vi "Timer Setup.vi"(5 "Timers":T1={"Timer"={"Sun"=FALSE, "Timer"=FALSE, "Altitude"=0.0, "Action Time"=55500.0, "Mon"=FALSE, "Tues"=TRUE, "Wed"=FALSE, "Thur"=FALSE, "Fri"=FALSE, "Sat"=FALSE, "Mode"=enum."Run"}, "Timer 2"={"Sun"=FALSE, "Timer"=FALSE, "Altitude"=0.0, "Action Time"=55560.0, "Mon"=FALSE, "Tues"=TRUE, "Wed"=FALSE, "Thur"=FALSE, "Fri"=FALSE, "Sat"=FALSE, "Mode"=enum."Stby"}, "Timer 3"={"Sun"=FALSE, "Timer"=FALSE, "Altitude"=0.0, "Action Time"=55680.0, "Mon"=FALSE, "Tues"=TRUE, "Wed"=FALSE, "Thur"=FALSE, "Fri"=FALSE, "Sat"=FALSE, "Mode"=enum."Run"}, "Timer 4"={"Sun"=FALSE, "Timer"=FALSE, "Altitude"=0.0, "Action Time"=55740.0, "Mon"=FALSE, "Tues"=TRUE, "Wed"=FALSE, "Thur"=FALSE, "Fri"=FALSE, "Sat"=FALSE, "Mode"=enum."Off"}} {"Timer 4"."Action Time" format="%<%H:%M>t"; "Timer 3"."Action Time" format="%<%H:%M>t"; "Timer 2"."Action Time" format="%<%H:%M>t"; "Timer"."Action Time" format="%<%H:%M>t"}) -> ()   [LabVIEW 2012]
uses:
  Type Defs/All Timers.ctl
  Type Defs/Timer Control.ctl
  Altitude/Altitude.xctl
  Type Defs/Action Time.ctl
  Mode Control/Mode.xctl
  Scheduler/Builder/Schedule Builder.lvclass
  Scheduler/Configuration Data/Task Data.lvclass
  MSR/Sequence Composition/Sequence Factory/Sequence Builder.lvclass/Sequence Builder.ctl
  Scheduler/Builder/Schedule Builder.lvclass/Schedule Builder.ctl
  MSR/Sequence Composition/SEQ/SEQ.lvclass
  Scheduler/Scheduler SEQ/Scheduler.lvclass
  Scheduler/Scheduler SEQ/Scheduler.lvclass/Scheduler.ctl
  Scheduler/Scheduler SEQ/Write DOW.vi
  MSR/Sequence Composition/Sequence Factory/Sequence Builder.lvclass
panel:
  in  "Tab Control":enum32{"Page 1", "Page 2"}(tab)
  out "Messages":string[](array[string])
  out "Timer.Mode":enum8{"Off", "Stby", "Hold", "Run"}(ring)
  out "Timer.Altitude":sgl
  # "1"
  # "1"
  # "1"
  # "1"
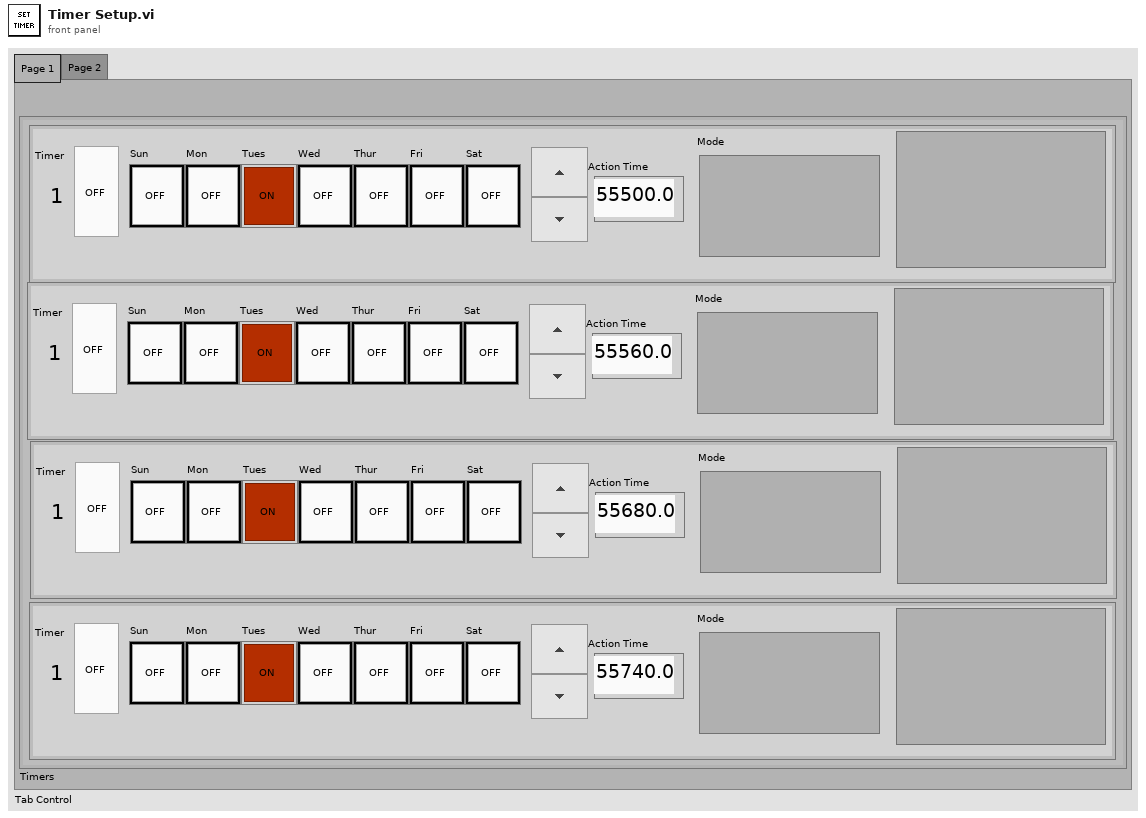
[diagram p1: front panel]
types:
  T1 = typedef "All Timers.ctl" = cluster{"Timer":T2, "Timer 2":T2, "Timer 3":T2, "Timer 4":T2}
  T2 = typedef "Timer Control.ctl" = cluster{"Sun":bool, "Timer":bool, "Altitude":sgl, "Action Time":T3, "Mon":bool, "Tues":bool, "Wed":bool, "Thur":bool, "Fri":bool, "Sat":bool, "Mode":enum8{"Off", "Stby", "Hold", "Run"}}
  T3 = typedef "Action Time.ctl" = dbl
  T4 = typedef "LVDateTimeRec.ctl" = cluster{"fractional second":dbl, "second":i32, "minute":i32, "hour":i32, "day of month":i32, "month":i32, "year":i32, "day of week":i32, "day of year":i32, "DST":i32}
  T5 = typedef "Mode Select.ctl" = enum8{"Off", "Stby", "Hold", "Run"}
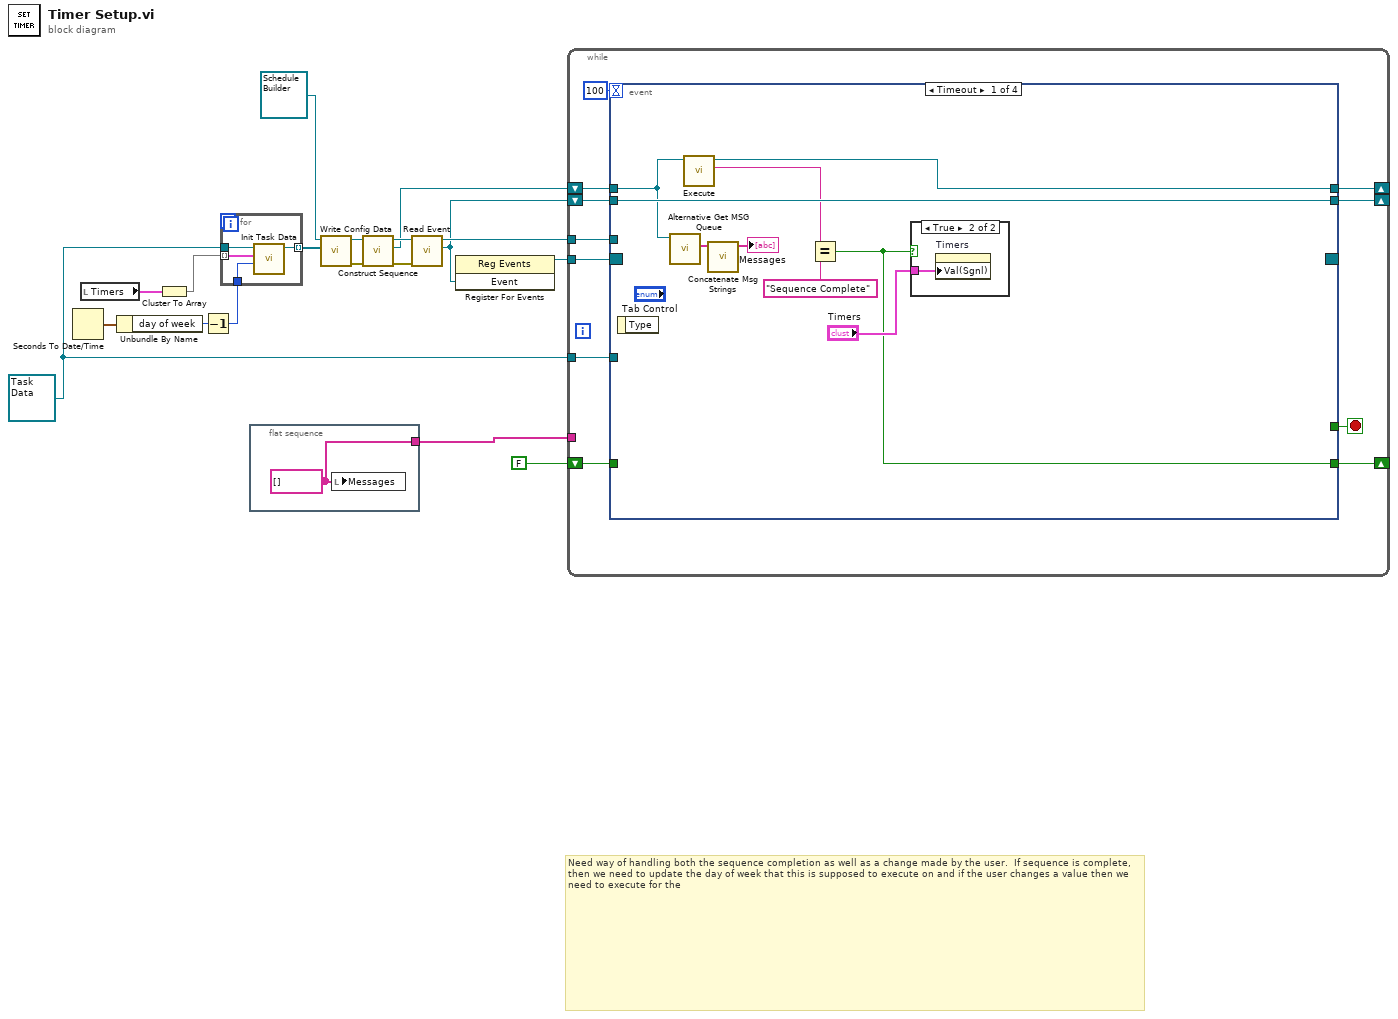
[diagram p0: block diagram]
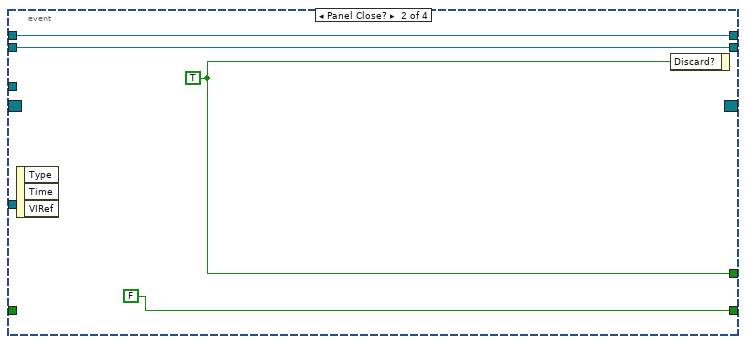
[diagram p3: hidden frame]
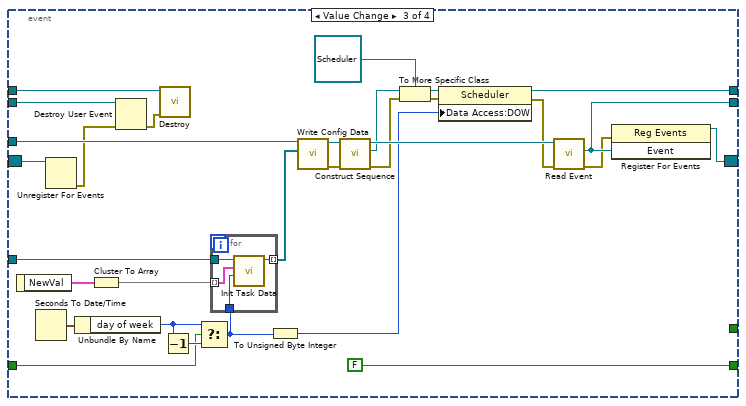
[diagram p4: hidden frame]
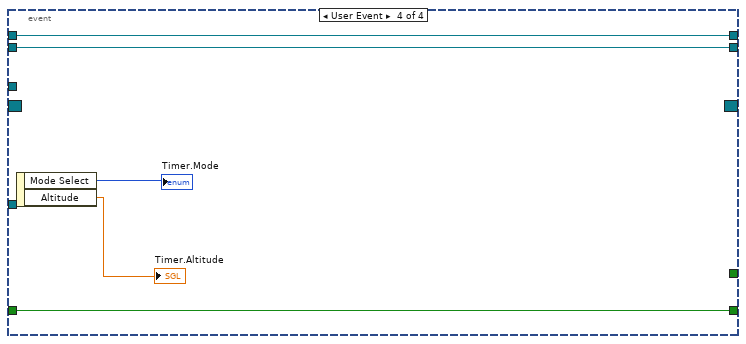
[diagram p5: hidden frame]
diagram:
  w8 = refnum<class "Task Data.lvclass"> refnum ("Task Data")
  # "Need way of handling both the sequence completion as well as a change made by the user.  If sequence is complete, then we need to update the day of week that this is supposed to execute on and if the user changes a value then we need to execute for the"
  n1 = Seconds To Date/Time() -> (date time rec=w4:T4)  [unwired: 2 in]
  n2 = local read "Timers"() -> (w13:T1)
  n3 = Unbundle By Name(w4) -> ("day of week"=w3:i32)
  n4 = Cluster To Array(cluster=w13) -> (array=w12:T2[])
  n5 = Decrement(x=w3) -> (x-1=w2:i32)
  n6 = for {
    tunnel: w12 -> [w22] mode=indexing
    tunnel: w8 -> [w21]
    tunnel: [w20] -> w11 mode=indexing
    tunnel: w2 -> [w19]
    n7 = call "Init Task Data.vi"("DOW"=w19, "Task In"=w22, "Task Data in"=w21) -> ("Task Data out"=w20:refnum<class "Task Data.lvclass">)  [unwired: 8 in]
  }
  n8 = flat-sequence {
    tunnel: [w23] -> w5
    frame #0 {
      w23 = string[] [] ("Messages")
      n9 = local write "Messages"(w23) -> ()
    }
  }
  n10 = call "Write Config Data.vi"("Config Data"=w11, "Sequence Builder in"=refnum<class "Schedule Builder.lvclass"> refnum ("Schedule Builder")) -> ("error out"=w16:errorcluster, "Sequence Builder out"=w17:refnum<class "Schedule Builder.lvclass">)  [unwired: 8 in]
  n11 = call-dynamic "Construct Sequence.vi"("error in"=w16, "Schedule Builder in"=w17) -> ("error out"=w14:errorcluster, "New Sequence"=w9:refnum<class "SEQ.lvclass">, "Schedule Builder out"=w15:refnum<class "Schedule Builder.lvclass">)  [unwired: 7 in]
  n12 = call "Read Event.vi"("error in (no error)"=w14, "Schedule Builder in"=w15) -> ("Event"=w6:refnum<user-event>, "Schedule Builder out"=w10:refnum<class "Schedule Builder.lvclass">)  [unwired: 7 in, 1 out]
  n13 = register-events(w6) -> (reference out=w7:refnum<event-registration>)  [unwired: 2 in, 1 out]
  n14 = while {
    tunnel: w10 -> [w32]
    shift-right: [w26] -> _
    shift-left: w9 -> [w31]
    tunnel: w8 -> [w30]
    tunnel: w7 -> [w29]
    shift-right: [w28] -> _
    shift-left: w6 -> [w27]
    tunnel: w5 -> [_]
    shift-right: [w24] -> _
    shift-left: FALSE -> [w25]
    stop <- w34 stop-if-true
    n15 = event shown="[0] Timeout" {
      selector: w29 -> [_ _ w68 _]
      dyn-events: [_ _ w69 _] -> _
      timeout: 100 -> [_ _ _ _]
      tunnel: [_ w48 _ _] -> w34
      tunnel: w32 -> [_ _ w71 _]
      tunnel: w31 -> [w40 w46 w78 w85]
      tunnel: w30 -> [_ _ w74 _]
      tunnel: [w43 w46 w49 w85] -> w26
      tunnel: [w42 w47 w67 w84] -> w28
      tunnel: w27 -> [w42 w47 w66 w84]
      tunnel: w25 -> [_ _ w50 w83]
      tunnel: [w35 FALSE FALSE w83] -> w24
      event Timeout {
        n16 = event-data() -> ()  [unwired: 1 in, 1 out]
        n17 = call "Alternative Get MSG Queue.vi"("SEQ in"=w40) -> ("seqMsg"=w41:string[])  [unwired: 9 in, 1 out]
        n18 = call-dynamic "Execute.vi"("SEQ in"=w40) -> ("MSG"=w38:string, "SEQ out"=w43:refnum<class "SEQ.lvclass">)  [unwired: 7 in, 2 out]
        n19 = call "Concatenate Msg Strings.vi"("StringsIn"=w41) -> ("StringsOut"=→"Messages":string[])  [unwired: 10 in]
        n20 = Equal?(x=w38, y="Sequence Complete" ("t")) -> (x = y?=w35:bool)
        n21 = case shown="True" w35 {
          tunnel: "Timers" -> [_ w44]
          frame False {
          }
          frame True {
            n22 = property on="Timers" class="Clust (strict)"("Val(Sgnl)"=w44) -> ()  [unwired: 2 in, 2 out]
          }
        }
      }
      event Panel Close? {
        w48 = TRUE
        n23 = event-data() -> ()  [unwired: 1 in, 3 out]
        n24 = event-data("Discard?"=w48) -> ()  [unwired: 1 in, 1 out]
      }
      event Value Change {
        n25 = event-data() -> ("NewVal"=w75:T1)  [unwired: 1 in]
        n26 = Seconds To Date/Time() -> (date time rec=w61:T4)  [unwired: 2 in]
        n27 = Unregister For Events(event registration refnum=w68) -> (error out=w65:errorcluster)  [unwired: 1 in]
        n28 = Unbundle By Name(w61) -> ("day of week"=w60:i32)
        n29 = Cluster To Array(cluster=w75) -> (array=w73:T2[])
        n30 = Destroy User Event(user event=w66, error in=w65) -> (error out=w64:errorcluster)
        n31 = call-dynamic "Destroy.vi"("error in"=w64, "SEQ in"=w78) -> ()  [unwired: 8 in, 2 out]
        n32 = Decrement(x=w60) -> (x-1=w59:i32)
        n33 = Select(t=w60, s=w50, f=w59) -> (s? t:f=w52:i32)
        n34 = for {
          tunnel: w73 -> [w82] mode=indexing
          tunnel: w74 -> [w81]
          tunnel: [w80] -> w72 mode=indexing
          tunnel: w52 -> [w79]
          n35 = call "Init Task Data.vi"("DOW"=w79, "Task In"=w82, "Task Data in"=w81) -> ("Task Data out"=w80:refnum<class "Task Data.lvclass">)  [unwired: 8 in]
        }
        n36 = To Unsigned Byte Integer(number=w52) -> (unsigned 8bit integer=w51:u8)
        n37 = call "Write Config Data.vi"("Config Data"=w72, "Sequence Builder in"=w71) -> ("error out"=w77:errorcluster, "Sequence Builder out"=w76:refnum<class "Schedule Builder.lvclass">)  [unwired: 8 in]
        n38 = call-dynamic "Construct Sequence.vi"("error in"=w77, "Schedule Builder in"=w76) -> ("error out"=w54:errorcluster, "New Sequence"=w58:refnum<class "SEQ.lvclass">, "Schedule Builder out"=w70:refnum<class "Schedule Builder.lvclass">)  [unwired: 7 in]
        n39 = To More Specific Class(target class=refnum<class "Scheduler.lvclass"> refnum ("Scheduler"), reference=w58, error in=w54) -> (specific class reference=w56:refnum<class "Scheduler.lvclass">, error out=w55:errorcluster)
        n40 = property class="Scheduler"(reference=w56, error in=w55, "Data Access:DOW"=w51) -> (reference out=w49:refnum<class "Scheduler.lvclass">, error out=w53:errorcluster)
        n41 = call "Read Event.vi"("error in (no error)"=w53, "Schedule Builder in"=w70) -> ("error out"=w63:errorcluster, "Event"=w67:refnum<user-event>)  [unwired: 7 in, 1 out]
        n42 = register-events(error in=w63, w67) -> (reference out=w69:refnum<event-registration>)  [unwired: 1 in, 1 out]
      }
      event User Event {
        n43 = event-data() -> ("Mode Select"=→"Timer.Mode":T5, "Altitude"=→"Timer.Altitude":sgl)  [unwired: 1 in]
      }
    }
  }
